vi "Remove Language.vi"(8 "error in (no error)":errorcluster, 10 "index":i32, 11 "LangFile in":refnum<class "Resource Data.lvclass">) -> (0 "error out":errorcluster, 3 "LangFile out":refnum<class "Resource Data.lvclass">)   [LabVIEW 2013, in "SET Project Data.lvlib" / "Resource Data.lvclass"]
uses:
  Resource Data.lvclass
  Resource Data.lvclass/Resource Data.ctl
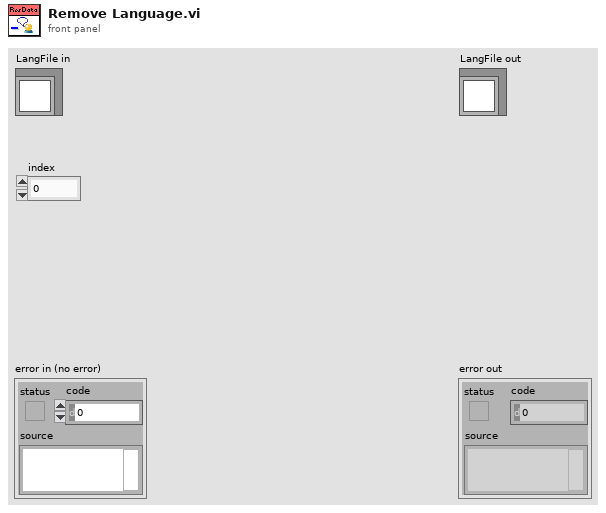
[diagram p1: front panel]
types:
  T1 = typedef "SET Project Data.lvlib/ProjFile_Language Entry.ctl" = cluster{"Tag":string, "Name":string, "Code Page":u16}
  T2 = typedef "SET Project Data.lvlib/ProjFile_Resource Entry.ctl" = cluster{"RID":string, "Tag":string, "Strings [] (UTF-16)":string[], "Shared?":bool}
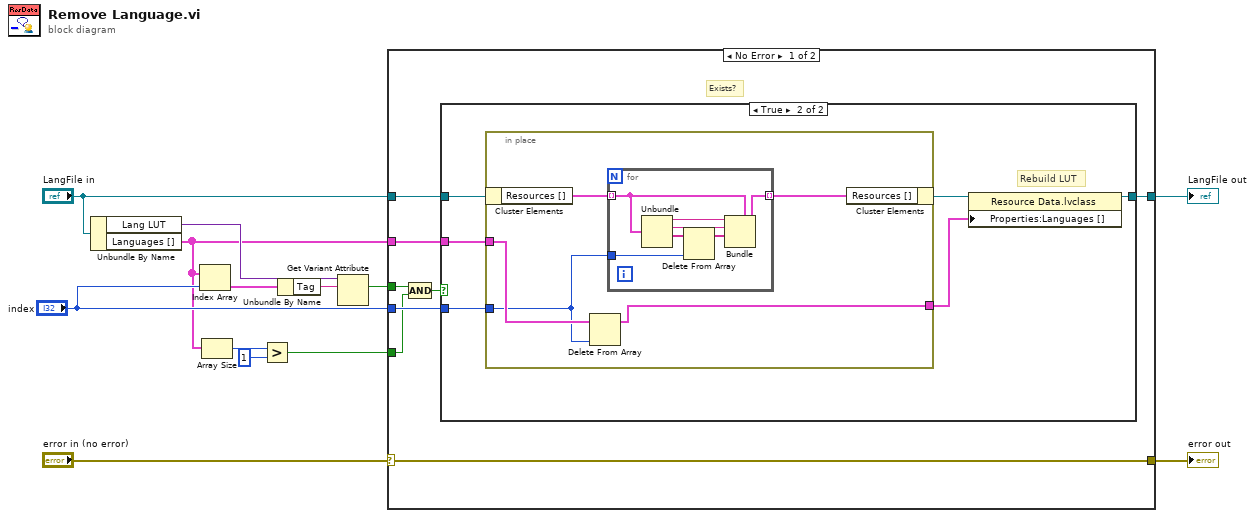
[diagram p0: block diagram]
diagram:
  n1 = Unbundle By Name("LangFile in") -> ("Lang LUT"=w8:variant, "Languages []"=w4:T1[])
  n2 = Index Array(array=w4, index="index") -> (element=w6:T1)
  n3 = Array Size(array=w4) -> (size(s)=w3:i32)
  n4 = Greater?(x=w3, y=1) -> (0:w1:bool)
  n5 = Unbundle By Name(w6) -> ("Tag"=w5:string)
  n6 = Get Variant Attribute(Variant=w8, name=w5) -> (found=w7:bool)  [unwired: 2 in, 3 out]
  n7 = case shown="No Error" "error in (no error)" {
    selector: "error in (no error)" -> [w21 w42]
    tunnel: [w21 w42] -> w12
    tunnel: [w19 w41] -> w11
    tunnel: "LangFile in" -> [w20 w41]
    tunnel: w7 -> [w16 _]
    tunnel: "index" -> [w18 _]
    tunnel: w4 -> [w17 _]
    tunnel: w1 -> [w15 _]
    frame No Error {
      # "Exists?"
      n8 = Compound Arithmetic op=AND(w16, w15) -> (w14:bool)
      n9 = case shown="True" w14 {
        tunnel: w20 -> [w22 w28]
        tunnel: [w22 w23] -> w19
        tunnel: w18 -> [_ w27]
        tunnel: w17 -> [_ w26]
        frame False {
        }
        frame True {
          # "Rebuild LUT"
          n10 = in-place {
            in-place-border: w27 -> [w30]
            in-place-border: w26 -> [w31]
            in-place-border: [w29] -> w24
            n11 = in-place-cluster #1(w28) -> ("Resources []"=w33:T2[])
            n12 = Delete From Array(array=w31, index=w30) -> (array with subset deleted=w29:T1[])  [unwired: 1 in, 1 out]
            n13 = for {
              tunnel: w33 -> [w35] mode=indexing
              tunnel: w30 -> [w36]
              tunnel: [w34] -> w32 mode=indexing
              n14 = Unbundle(w35) -> ("RID"=w40:string, "Tag"=w39:string, "Strings [] (UTF-16)"=w38:string[])  [unwired: 1 out]
              n15 = Delete From Array(array=w38, index=w36) -> (array with subset deleted=w37:string[])  [unwired: 1 in, 1 out]
              n16 = Bundle(cluster=w35, "RID"=w40, "Tag"=w39, "Strings [] (UTF-16)"=w37) -> (w34:T2)  [unwired: 1 in]
            }
            n17 = in-place-cluster #1("Resources []"=w32) -> (w25:refnum<class "Resource Data.lvclass">)
          }
          n18 = property class="Resource Data.lvclass"(reference=w25, "Properties:Languages []"=w24) -> (reference out=w23:refnum<class "Resource Data.lvclass">)  [unwired: 1 in, 1 out]
        }
      }
    }
    frame Error {
    }
  }
  "error out" <- w12
  "LangFile out" <- w11
